vi "determineTargetType.vi"(8 "error in (no error)":errorcluster, 10 "childAttributes":T1[](array[typedef])) -> (0 "error out":errorcluster, 3 "Target.lvclass":refnum<class "Target.lvclass">)   [LabVIEW 2022 SP3, in "TCSDataDefinitions.lvlib" / "TCSCommand.lvlib" / "TargetConfiguration.lvlib" / "Target.lvlib" / "Target.lvclass"]
uses:
  Target/Target.lvclass
  <userlib>/Common/XML/Typedefs/AttributeElements.ctl
  FixedTarget/RADecTarget/RADecTarget.lvclass
  C:/Development/rimas/RIMAS/TCS/TCS_external_interfaces/TCSDataDefinitions/TCSCommand/TargetConfiguration/Target/Target/Target.lvclass
  FixedTarget/AzElTarget/AzElTarget.lvclass
  Ephemeris/Ephemeris.lvclass
  Planet/Planet.lvclass
  <userlib>/Common/XML/XML.lvlib
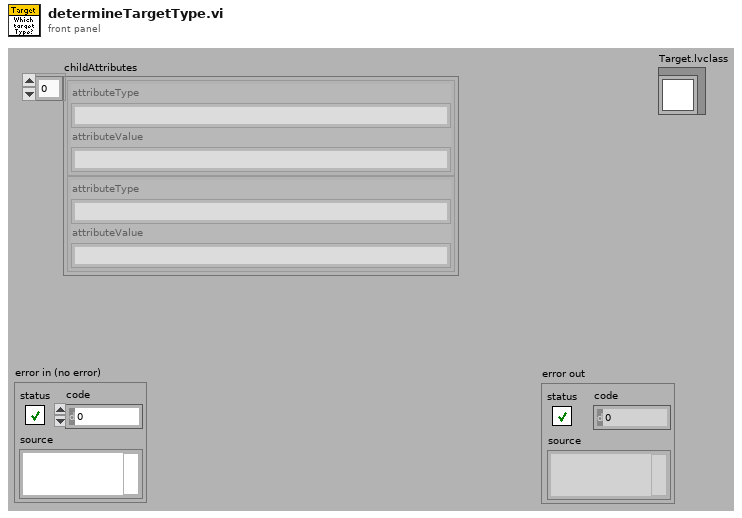
[diagram p1: front panel]
types:
  T1 = typedef "XML.lvlib/AttributeElements.ctl" = cluster{"attributeType":string, "attributeValue":string}
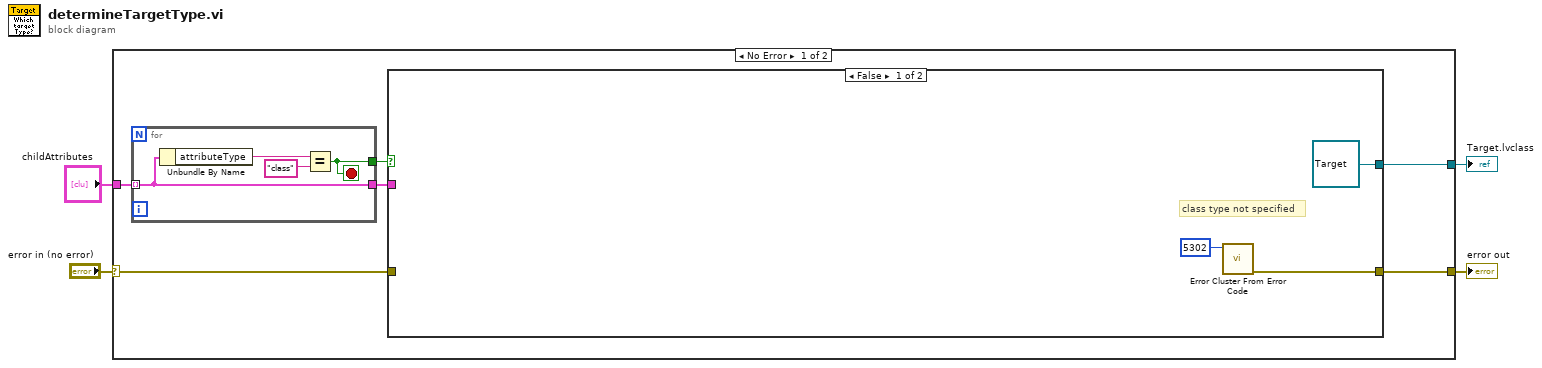
[diagram p0: block diagram]
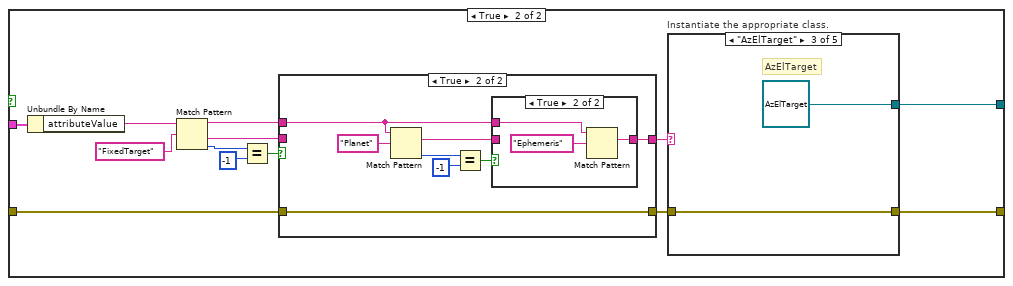
[diagram p2: hidden frame]
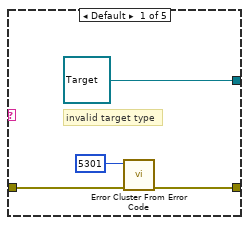
[diagram p3: hidden frame]
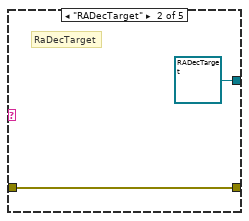
[diagram p4: hidden frame]
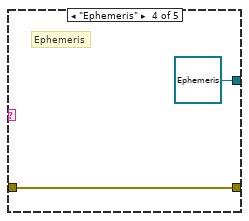
[diagram p5: hidden frame]
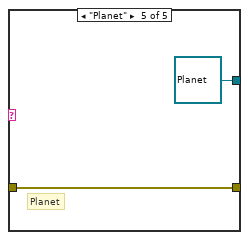
[diagram p6: hidden frame]
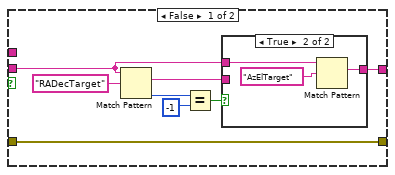
[diagram p7: hidden frame]
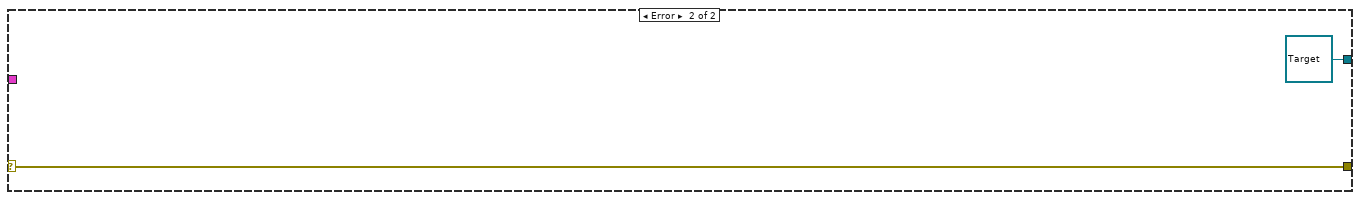
[diagram p10: hidden frame]
diagram:
  n1 = case shown="No Error" "error in (no error)" {
    selector: "error in (no error)" -> [w10 w67]
    tunnel: [w9 refnum<class "Target.lvclass"> refnum ("Target.lvclass")] -> w3
    tunnel: "childAttributes" -> [w7 _]
    tunnel: [w8 w67] -> w1
    frame No Error {
      n2 = for {
        tunnel: w7 -> [w64] mode=indexing
        tunnel: [w64] -> w6
        tunnel: [w63] -> w5
        stop <- w63 stop-if-true
        n3 = Unbundle By Name(w64) -> ("attributeType"=w65:string)
        n4 = Equal?(x=w65, y="class") -> (x = y?=w63:bool)
      }
      n5 = case shown="False" w5 {
        tunnel: w10 -> [_ w26]
        tunnel: [refnum<class "Target.lvclass"> refnum ("Target.lvclass") w25] -> w9
        tunnel: [w11 w14] -> w8
        tunnel: w6 -> [_ w23]
        frame False {
          # "class type not specified"
          n6 = call <vilib>:"Error Cluster From Error Code.vi"("error code (0)"=5302 ("code")) -> ("error out"=w11:errorcluster)  [unwired: 8 in]
        }
        frame True {
          n7 = Unbundle By Name(w23) -> ("attributeValue"=w24:string)
          n8 = Match Pattern(string=w24, regular expression="FixedTarget") -> (before substring=w15:string, after substring=w18:string, offset past match=w21:i32)  [unwired: 1 in, 1 out]
          n9 = Equal?(x=w21, y=-1) -> (x = y?=w19:bool)
          n10 = case shown="True" w19 {
            tunnel: w26 -> [w39 w58]
            tunnel: [w39 w58] -> w17
            tunnel: w18 -> [w45 _]
            tunnel: [w40 w52] -> w16
            tunnel: w15 -> [_ w51]
            frame False {
              n11 = Match Pattern(string=w45, regular expression="RADecTarget") -> (match substring=w41:string, offset past match=w44:i32)  [unwired: 1 in, 2 out]
              n12 = Equal?(x=w44, y=-1) -> (x = y?=w42:bool)
              n13 = case shown="True" w42 {
                tunnel: w45 -> [_ w49]
                tunnel: w41 -> [w47 _]
                tunnel: [w47 w48] -> w40
                frame False {
                }
                frame True {
                  n14 = Match Pattern(string=w49, regular expression="AzElTarget") -> (match substring=w48:string)  [unwired: 1 in, 3 out]
                }
              }
            }
            frame True {
              n15 = Match Pattern(string=w51, regular expression="Planet") -> (match substring=w53:string, offset past match=w56:i32)  [unwired: 1 in, 2 out]
              n16 = Equal?(x=w56, y=-1) -> (x = y?=w54:bool)
              n17 = case shown="True" w54 {
                tunnel: w51 -> [_ w61]
                tunnel: w53 -> [w59 _]
                tunnel: [w59 w60] -> w52
                frame False {
                }
                frame True {
                  n18 = Match Pattern(string=w61, regular expression="Ephemeris") -> (match substring=w60:string)  [unwired: 1 in, 3 out]
                }
              }
            }
          }
          n19 = case "Instantiate the appropriate class." shown="\"AzElTarget\"" w16 {
            tunnel: [w28 w31 w33 w35 w37] -> w14
            tunnel: [refnum<class "Target.lvclass"> refnum ("Target.lvclass") refnum<class "RADecTarget.lvclass"> refnum ("RADecTarget.lvclass") refnum<class "AzElTarget.lvclass"> refnum ("AzElTarget.lvclass") refnum<class "Ephemeris.lvclass"> refnum ("Ephemeris.lvclass") refnum<class "Planet.lvclass"> refnum ("Planet.lvclass")] -> w25
            tunnel: w17 -> [w27 w31 w33 w35 w37]
            frame Default {
              # "invalid target type"
              n20 = call <vilib>:"Error Cluster From Error Code.vi"("error in (no error)"=w27, "error code (0)"=5301 ("code")) -> ("error out"=w28:errorcluster)  [unwired: 7 in]
            }
            frame "RADecTarget" {
              # "RaDecTarget"
            }
            frame "AzElTarget" {
              # "AzElTarget"
            }
            frame "Ephemeris" {
              # "Ephemeris"
            }
            frame "Planet" {
              # "Planet"
            }
          }
        }
      }
    }
    frame Error {
    }
  }
  "error out" <- w1
  "Target.lvclass" <- w3
